vi "misc-1.vi"() -> ()   [LabVIEW 2022 SP3]
panel:
  in  "Tab Control":enum32{"Page 1", "Page 2", "Page 3"}(tab)
  out "Waveform Chart":dbl(graph)
  out "Waveform Graph":dbl[](graph)
  out "XY Graph":cluster{"Y":dbl[], "Y":dbl[]}[](graph)
  in  "[ESC]":bool
  out "error constant":errorcluster={"status"=FALSE, "code"=10, "source"="Rahi ghalta"}
  out "Appended Array":dbl[](array[numeric])
  out "Num Value":dbl
  out "Boolean":bool
  out "output cluster":cluster{"Num Value Out":dbl, "aa":bool}
  in  "Cluster":cluster{"Num Value In":dbl, "aa":bool}
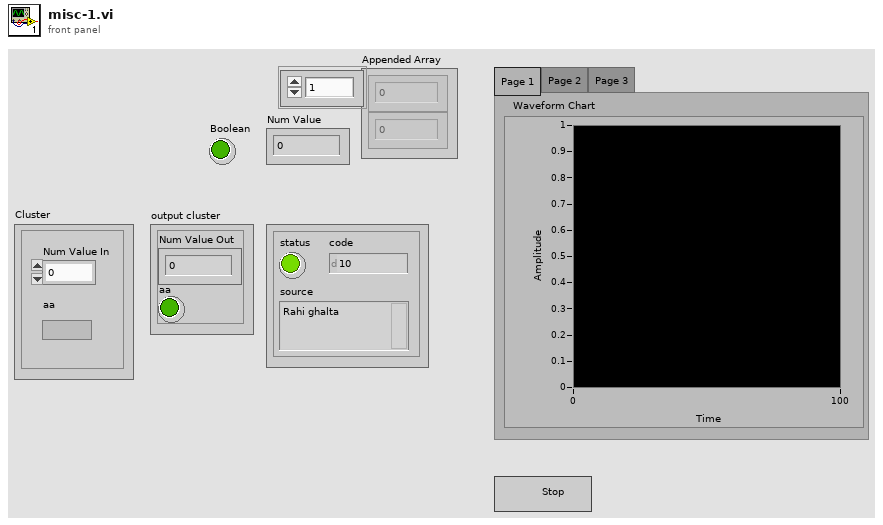
[diagram p1: front panel]
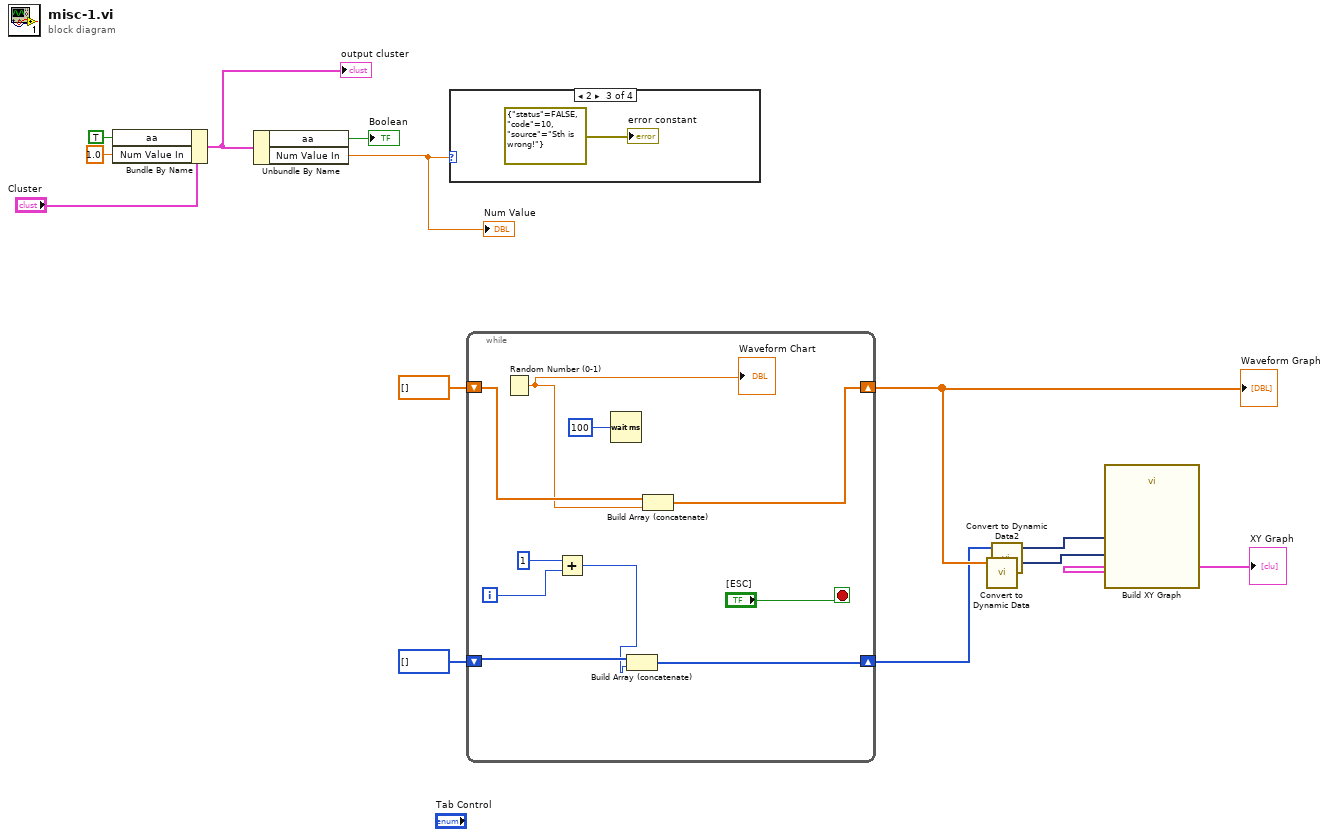
[diagram p0: block diagram]
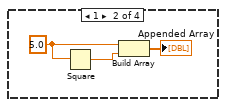
[diagram p3: hidden frame]
diagram:
  n1 = Bundle By Name(cluster="Cluster", "aa"=TRUE, "Num Value In"=1.0) -> (w11:cluster{"Num Value In":dbl, "aa":bool})
  "output cluster" <- w11
  n2 = Unbundle By Name(w11) -> ("aa"=→"Boolean":bool, "Num Value In"=w10:dbl)
  "Num Value" <- w10
  n3 = case shown="2" w10 {
    frame 0, Default {
    }
    frame 1 {
      w15 = 5.0 ("element")
      n4 = Square(x=w15) -> (x^2=w16:dbl)
      n5 = Build Array(w15, w16) -> (→"Appended Array":dbl[])
    }
    frame 2 {
      "error constant" <- errorcluster {"status"=FALSE, "code"=10, "source"="Sth is wrong!"} ("error constant")
    }
    frame 3 {
    }
  }
  n6 = while {
    shift-right: [w26] -> w7
    shift-left: dbl[] [] -> [w25]
    shift-right: [w21] -> w5
    shift-left: i32[] [] -> [w22]
    i -> [w24]
    stop <- "[ESC]" stop-if-true
    n7 = Random Number (0-1)() -> (number: 0 to 1=w20:dbl)
    "Waveform Chart" <- w20
    n8 = Add(x=1, y=w24) -> (x+y=w19:i32)
    n9 = Wait (ms)(milliseconds to wait=u32 100) -> ()  [unwired: 1 out]
    n10 = Build Array (concatenate)(w22, w19) -> (w21:i32[])
    n11 = Build Array (concatenate)(w25, w20) -> (w26:dbl[])
  }
  "Waveform Graph" <- w7
  n12 = call "Convert to Dynamic Data"("Array"=w7) -> ("Dynamic Data Type"=w6:dynamicdata)  [unwired: 3 in]
  n13 = call "Convert to Dynamic Data2"("Array"=w5) -> ("Dynamic Data Type"=w4:dynamicdata)  [unwired: 3 in]
  n14 = call "Build XY Graph"("Y Input"=w6, "X Input"=w4) -> ("XY Graph"=→"XY Graph":cluster{"Y":dbl[], "Y":dbl[]}[])  [unwired: 3 in, 6 out]
